vi "FIFOLifetime_HH.vi"(0 "input rawdata":T1, 1 "range":cluster{"x0":dbl, "x1":dbl} {"x1" format="%.2f"; "x0" format="%.2f"}, 2 "rebinning":dbl=1.0 min=1.0 max=4000.0 step=1.0, 4 "channel count":dbl) -> (5 "lifetime histograms":u32[][](array[numeric]))   [LabVIEW 2009]
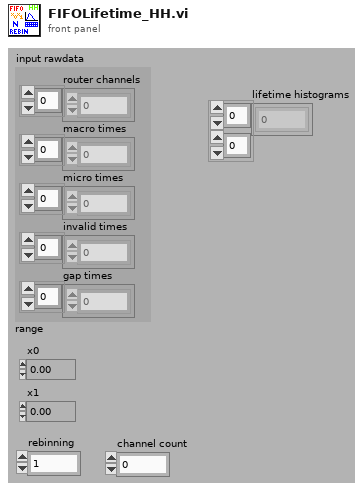
[diagram p1: front panel]
types:
  T1 = cluster{"router channels":i8[], "macro times":u32[], "micro times":u16[], "invalid times":u32[], "gap times":u32[]}
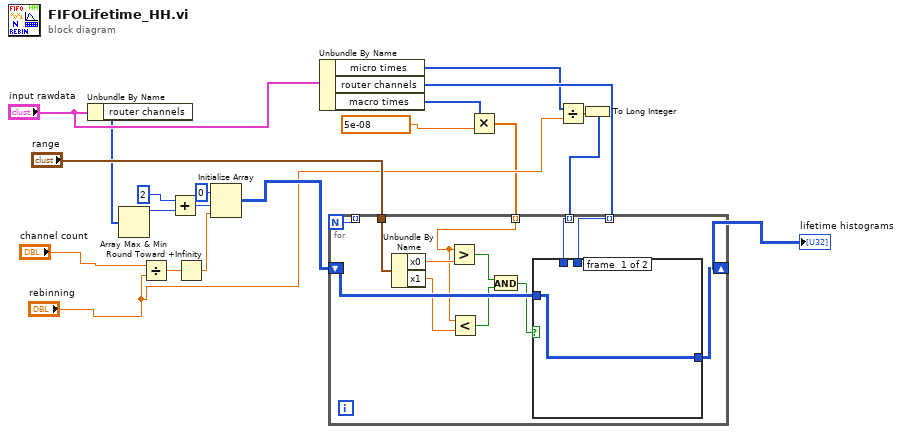
[diagram p0: block diagram]
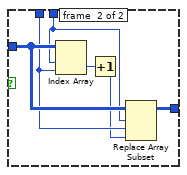
[diagram p2: hidden frame]
diagram:
  n1 = Unbundle By Name("input rawdata") -> ("router channels"=w12:i8[])
  n2 = Array Max & Min(array=w12) -> (max value=w16:i8)  [unwired: 3 out]
  n3 = Divide(x="channel count", y="rebinning") -> (x/y=w13:dbl)
  n4 = Add(x=u8 2, y=w16) -> (x+y=w15:u8)
  n5 = Round Toward +Infinity(x=w13) -> (ceil(x): smallest int >= x=w9:dbl)
  n6 = Initialize Array(0 ("element"), w15, w9) -> (w18:i32[][])
  n7 = Unbundle By Name("input rawdata") -> ("micro times"=w3:u16[], "router channels"=w7:i8[], "macro times"=w6:u32[])
  n8 = Multiply(x=w6, y=5e-08) -> (x*y=w1:dbl[])
  n9 = Divide(x=w3, y="rebinning") -> (x/y=w5:dbl[])
  n10 = To Long Integer(number=w5) -> (32bit integer=w4:i32[])
  n11 = for {
    N -> [w21]
    tunnel: w4 -> [w30] mode=indexing
    shift-right: [w29] -> w10
    shift-left: w18 -> [w32]
    tunnel: w7 -> [w31] mode=indexing
    tunnel: w1 -> [w25] mode=indexing
    tunnel: "range" -> [w28]
    tunnel: [w21] -> _ mode=indexing
    n12 = Unbundle By Name(w28) -> ("x0"=w27:dbl, "x1"=w26:dbl)
    n13 = Greater?(x=w25, y=w27) -> (0:w24:bool)
    n14 = Less?(x=w25, y=w26) -> (x < y?=w23:bool)
    n15 = And(x=w24, y=w23) -> (x .and. y?=w22:bool)
    n16 = case shown="True" w22 {
      tunnel: w32 -> [w33 w38]
      tunnel: w31 -> [_ w34]
      tunnel: w30 -> [_ w37]
      tunnel: [w33 w35] -> w29
      frame #0 {
      }
      frame #1 {
        n17 = Index Array(array=w38, index (row)=w34, index (col)=w37) -> (element=w39:i32)
        n18 = Increment(x=w39) -> (x+1=w36:i32)
        n19 = Replace Array Subset(array=w38, new element=w36, index (row)=w34, index (col)=w37) -> (w35:i32[][])
      }
    }
  }
  "lifetime histograms" <- w10
